vi "Server2.vi"() -> ()   [LabVIEW 2015]
panel:
  in  "Sampling Frequency (Hz)":dbl format="%#_13g"
  out "Wavelength Data":string="Wavelength Data"
  in  "Wavelength Data":string="Wavelength Data"
  out "Error out":errorcluster
  in  "Stop Sending":bool
  out "Error out 2":errorcluster
  out "Received Message":string
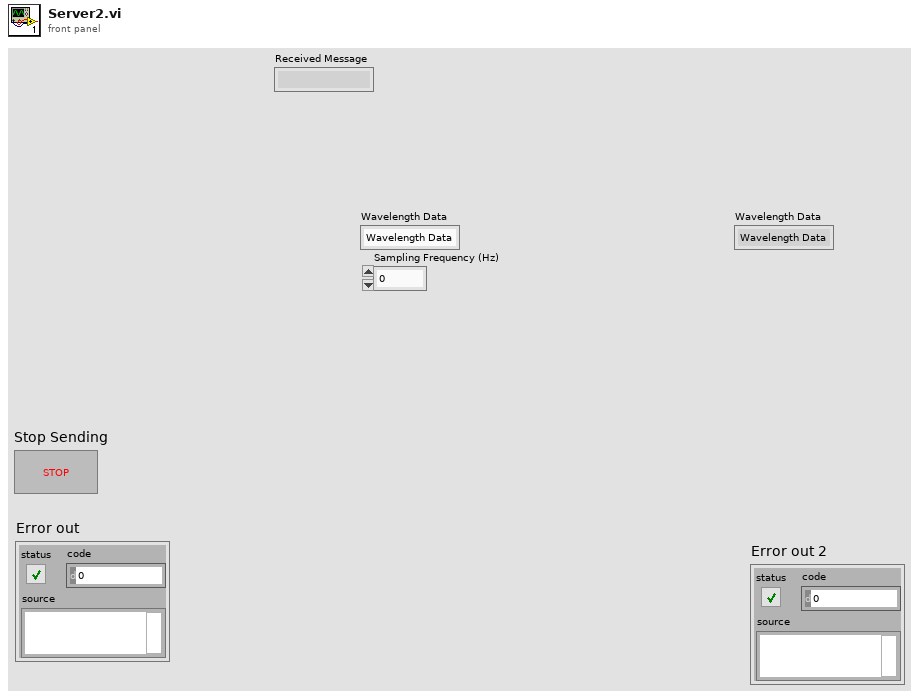
[diagram p1: front panel]
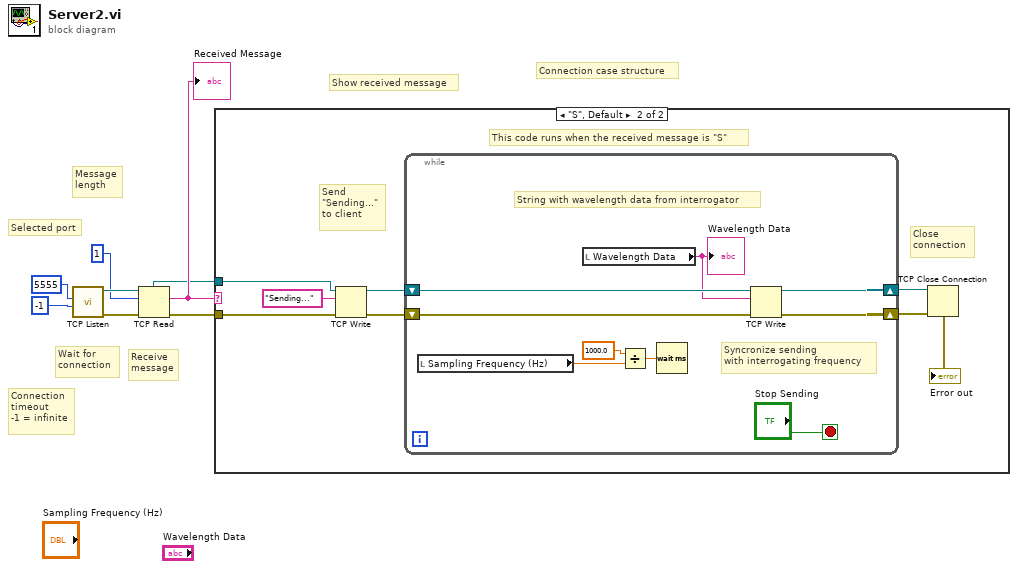
[diagram p0: block diagram]
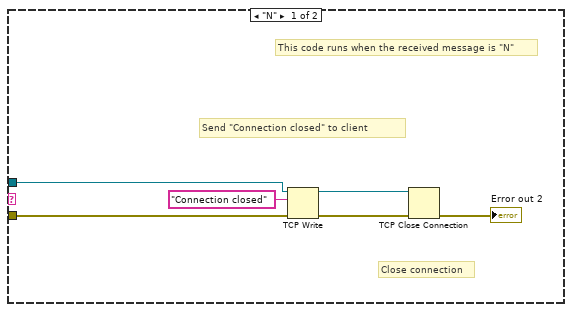
[diagram p2: hidden frame]
diagram:
  # "Connection case structure"
  # "Receive\nmessage"
  # "Wait for\nconnection"
  # "Message\nlength"
  # "Connection\ntimeout\n-1 = infinite"
  # "Selected port"
  # "Show received message"
  n1 = call <vilib>:"TCP Listen.vi"("timeout ms (wait forever: -1)"=-1 ("Timeout [ms]\n (wait forever: -1)"), "port"=u16 5555 ("Port")) -> ("error out"=w5:errorcluster, "connection ID"=w6:refnum<k5>)  [unwired: 5 in, 3 out]
  n2 = TCP Read(connection ID=w6, bytes to read=1, error in (no error)=w5) -> (connection ID out=w2:refnum<k5>, data out=w3:string, error out=w1:errorcluster)  [unwired: 2 in]
  "Received Message" <- w3
  n3 = case shown="\"S\", Default" w3 {
    tunnel: w2 -> [w13 w19]
    tunnel: w1 -> [w12 w17]
    frame "N" {
      # "Close connection"
      # "Send \"Connection closed\" to client"
      # "This code runs when the received message is \"N\""
      n4 = TCP Write(connection ID=w13, data in="Connection closed", error in (no error)=w12) -> (connection ID out=w9:refnum<k5>, error out=w10:errorcluster)  [unwired: 1 in, 1 out]
      n5 = TCP Close Connection(connection ID=w9, error in (no error)=w10) -> (error out=→"Error out 2":errorcluster)  [unwired: 1 in, 1 out]
    }
    frame "S", Default {
      # "Close \nconnection"
      # "This code runs when the received message is \"S\""
      # "Send\n\"Sending...\"\nto client"
      n6 = TCP Write(connection ID=w19, data in="Sending...", error in (no error)=w17) -> (connection ID out=w18:refnum<k5>, error out=w16:errorcluster)  [unwired: 1 in, 1 out]
      n7 = while {
        shift-right: [w30] -> w21
        shift-left: w18 -> [w31]
        shift-right: [w28] -> w20
        shift-left: w16 -> [w29]
        stop <- "Stop Sending" stop-if-true
        # "Syncronize sending\nwith interrogating frequency"
        # "String with wavelength data from interrogator"
        n8 = local read "Sampling Frequency (Hz)"() -> (w25:dbl)
        n9 = local read "Wavelength Data"() -> (w26:string)
        "Wavelength Data" <- w26
        n10 = Divide(x=1000.0, y=w25) -> (x/y=w23:dbl)
        n11 = Wait (ms)(milliseconds to wait=w23) -> ()  [unwired: 1 out]
        n12 = TCP Write(connection ID=w31, data in=w26, error in (no error)=w29) -> (connection ID out=w30:refnum<k5>, error out=w28:errorcluster)  [unwired: 1 in, 1 out]
      }
      n13 = TCP Close Connection(connection ID=w21, error in (no error)=w20) -> (error out=→"Error out":errorcluster)  [unwired: 1 in, 1 out]
    }
  }
